vi "Loop_ACT.vi"() -> ()   [LabVIEW 2017, in "TemplateActuator.lvlib"]
uses:
  TemplateActuator.lvlib
  _SOURCE2018_Master/_SHARE ALL/Global Share All/Global_STOP.vi
  Global_SM Write_Data Out.vi
  Global_ACT Write_Data Out.vi
panel:
  out "Output Data":dbl
  out "Input Data":dbl
  out "Cycle Time (S)":dbl format="%.3g"
  in  "Target Time(ms)":u32=50
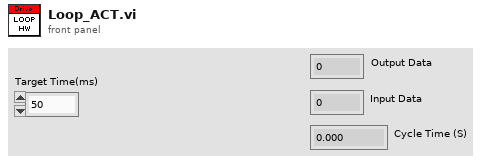
[diagram p1: front panel]
types:
  T1 = cluster{"Actuator Ref Data":cluster{i32}, " Actuator Output":dbl, "Actuator Input":dbl, "Target Time(ms)":u32, "Current Time":timestamp, "Previous Time":timestamp, "Cycle Time (S)":dbl}
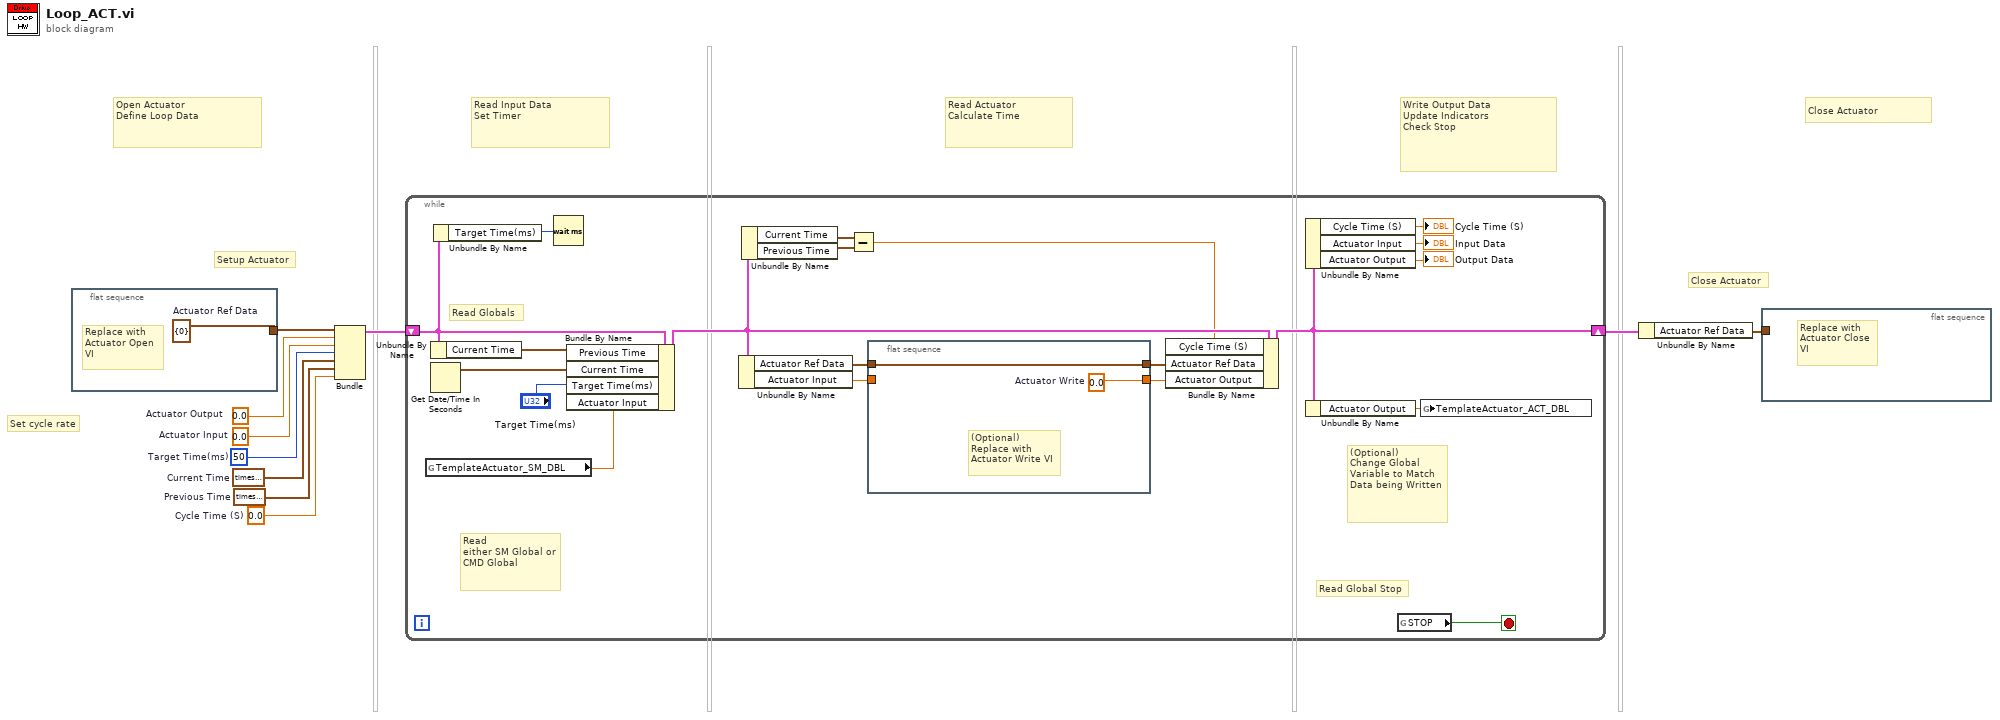
[diagram p0: block diagram]
diagram:
  w1 = 0.0  # Cycle Time (S)
  w10 = timestamp(0 s since 1904-01-01)  # Previous Time
  w9 = timestamp(0 s since 1904-01-01)  # Current Time
  w8 = u32 50  # Target Time(ms)
  w6 = 0.0  # Actuator Input
  w4 = 0.0  # Actuator Output
  # "Close Actuator"
  # "Write Output Data\nUpdate Indicators\nCheck Stop"
  # "Read Actuator\nCalculate Time"
  # "Read Input Data\nSet Timer"
  # "Open Actuator\nDefine Loop Data"
  # "Set cycle rate"
  # "Close Actuator"
  # "Setup Actuator"
  n1 = flat-sequence {
    tunnel: [w11] -> w3
    frame #0 {
      w11 = cluster{i32} {0}  # Actuator Ref Data
      # "Replace with \nActuator Open\nVI"
    }
  }
  n2 = Bundle("Actuator Ref Data"=w3, "Actuator Output"=w4, "Actuator Input"=w6, "Target Time(ms)"=w8, "Current Time"=w9, "Previous Time"=w10, "Cycle Time (S)"=w1) -> (w5:T1)  [unwired: 1 in]
  n3 = while {
    shift-right: [w18] -> w2
    shift-left: w5 -> [w20]
    stop <- w31 stop-if-true
    # "(Optional)\nChange Global\nVariable to Match\nData being Written"
    # "Read\neither SM Global or CMD Global"
    # "Read Globals"
    # "Read Global Stop"
    n4 = global read "Global_SM Write_Data Out.vi" "TemplateActuator_SM_DBL"() -> (w12:dbl)
    n5 = Unbundle By Name(w20) -> ("Current Time"=w25:timestamp)
    n6 = Get Date/Time In Seconds() -> (seconds since 1Jan1904=w26:timestamp)
    n7 = Unbundle By Name(w20) -> ("Target Time(ms)"=w19:u32)
    n8 = Wait (ms)(milliseconds to wait=w19) -> ()  [unwired: 1 out]
    n9 = Bundle By Name(cluster=w20, "Previous Time"=w25, "Current Time"=w26, "Target Time(ms)"="Target Time(ms)", "Actuator Input"=w12) -> (w21:T1)
    n10 = Unbundle By Name(w21) -> ("Actuator Ref Data"=w30:cluster{i32}, "Actuator Input"=w28:dbl)
    n11 = Unbundle By Name(w21) -> ("Current Time"=w24:timestamp, "Previous Time"=w23:timestamp)
    n12 = Subtract(x=w24, y=w23) -> (x-y=w14:dbl)
    n13 = flat-sequence {
      tunnel: w30 -> [w33]
      tunnel: [w33] -> w29
      tunnel: [w32] -> w27
      tunnel: w28 -> [_]
      frame #0 {
        w32 = 0.0  # Actuator Write
        # "(Optional)\nReplace with\nActuator Write VI"
      }
    }
    n14 = Bundle By Name(cluster=w21, "Cycle Time (S)"=w14, "Actuator Ref Data"=w29, "Actuator Output"=w27) -> (w18:T1)
    n15 = Unbundle By Name(w18) -> ("Cycle Time (S)"=→"Cycle Time (S)":dbl, "Actuator Input"=→"Input Data":dbl, "Actuator Output"=→"Output Data":dbl)
    n16 = Unbundle By Name(w18) -> ("Actuator Output"=w13:dbl)
    n17 = global read "Global_STOP.vi" "STOP"() -> (w31:bool)
    n18 = global write "Global_ACT Write_Data Out.vi" "TemplateActuator_ACT_DBL"(w13) -> ()
  }
  n19 = Unbundle By Name(w2) -> ("Actuator Ref Data"=w7:cluster{i32})
  n20 = flat-sequence {
    tunnel: w7 -> [_]
    frame #0 {
      # "Replace with \nActuator Close\nVI"
    }
  }
